vi "ParameterUpdate.vi"(5 "模式":T1(ring)=enum."updatesave", 7 "productsName":string, 8 "limitL":dbl=nan, 9 "limitH":dbl=nan, 10 "vaule":dbl=nan, 11 "parameterName":string) -> ()   [LabVIEW 2012]
uses:
  <vilib>/Utility/VariantDataType/Type.ctl
  <vilib>/Utility/VariantDataType/VariantType.lvlib
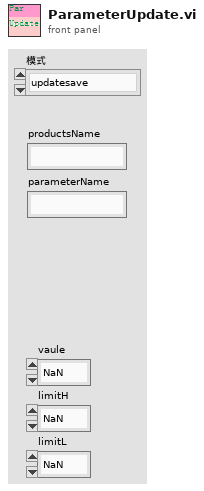
[diagram p1: front panel]
types:
  T1 = enum16{"updatedata", "updatesave", "updateresult", "updateresultempty"}
  T2 = typedef "VariantType.lvlib/Type.ctl" = enum8{"Invalid Type", "Void", "I8", "I16", "I32", "I64", "U8", "U16", "U32", "U64", "Single Float", "Double Float", "Extended Float", "Single Complex", "Double Complex", "Extended Complex", "Enum U8", "Enum U16", "Enum U32", "Enum U64", "Single Float With Unit", "Double Float With Unit", "Extended Float With Unit", "Single Complex with Unit", "Double Complex with Unit", "Extended Complex with Unit", "Boolean", "String", "Path", "Picture", "Tag", "Array", "Cluster", "Variant", "LV Variant", "Waveform", "Timestamp", "Digital Waveform", "Digital Data", "ExpressData", "Refnum", "External Data", "VI", "Poly VI", "LabVIEW Class Instance", "Fixed Point"}
  T3 = enum16{"selectdata", "selectsave", "selectlist", "selectshow"}
  T4 = cluster{"Type Enum":T2, "标签.文本":string, "productsName":string}
  T5 = cluster{"Type Enum":T2, "标签.文本":string, "productsName":string}[]
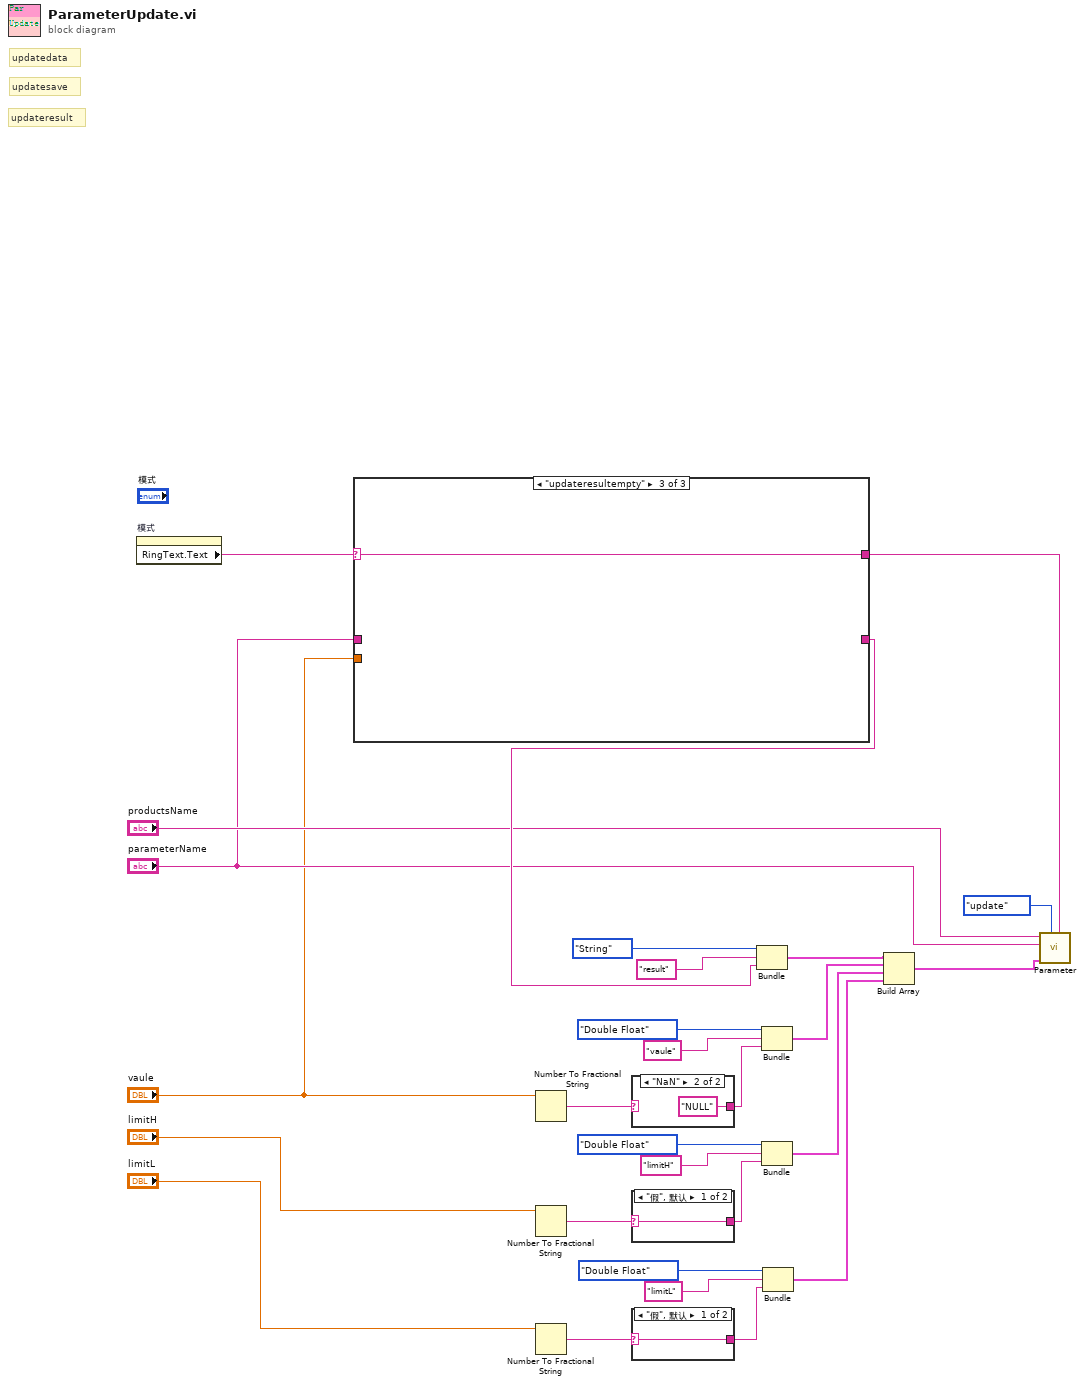
[diagram p0: block diagram]
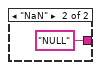
[diagram p3: hidden frame]
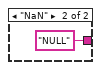
[diagram p4: hidden frame]
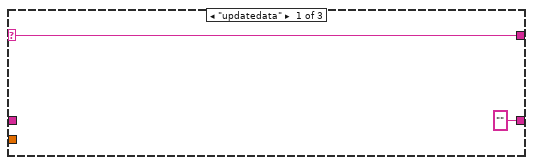
[diagram p5: hidden frame]
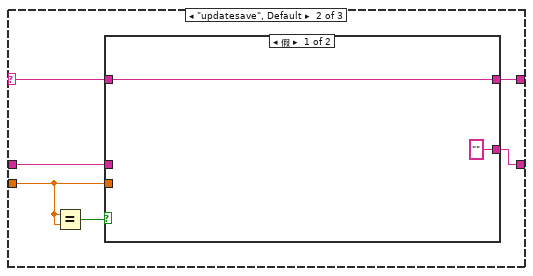
[diagram p6: hidden frame]
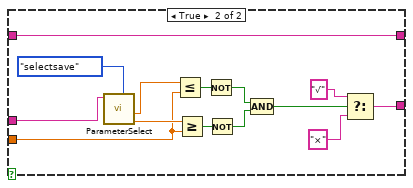
[diagram p7: hidden frame]
diagram:
  # "updatedata"
  # "updatesave"
  # "updateresult"
  n1 = property on="模式" class="Enum (严格)"() -> ("RingText.Text"=w28:string)  [unwired: 2 in, 2 out]
  n2 = case shown="\"updateresultempty\"" w28 {
    selector: w28 -> [w30 w34 w53]
    tunnel: "parameterName" -> [_ w36 _]
    tunnel: ["" ("productsName") w35 _] -> w12
    tunnel: [w30 w33 w53] -> w13
    tunnel: "vaule" -> [_ w31 _]
    frame "updatedata" {
    }
    frame "updatesave", Default {
      n3 = Equal?(x=w31, y=w31) -> (x = y?=w32:bool)
      n4 = case shown="假" w32 {
        tunnel: w36 -> [_ w52]
        tunnel: ["" ("productsName") w48] -> w35
        tunnel: w31 -> [_ w41]
        tunnel: w34 -> [w38 w39]
        tunnel: [w38 w39] -> w33
        frame False {
        }
        frame True {
          n5 = call "ParameterSelect.vi"("模式"=T3."selectsave", "parameterName"=w52) -> ("limitL"=w43:dbl, "limitH"=w42:dbl)  [unwired: 4 in, 4 out]
          n6 = Less Or Equal?(x=w42, y=w41) -> (x <= y?=w47:bool)
          n7 = Greater Or Equal?(x=w43, y=w41) -> (x >= y?=w45:bool)
          n8 = Not(x=w47) -> (.not. x?=w46:bool)
          n9 = Not(x=w45) -> (.not. x?=w44:bool)
          n10 = Compound Arithmetic op=AND(w46, w44) -> (w40:bool)
          n11 = Select(t="√" ("productsName"), s=w40, f="×" ("productsName")) -> (s? t:f=w48:string)
        }
      }
    }
    frame "updateresultempty" {
    }
  }
  n12 = Number To Fractional String(number="vaule") -> (F-format string=w8:string)  [unwired: 3 in]
  n13 = Number To Fractional String(number="limitH") -> (F-format string=w17:string)  [unwired: 3 in]
  n14 = Number To Fractional String(number="limitL") -> (F-format string=w19:string)  [unwired: 3 in]
  n15 = case shown="\"NaN\"" w8 {
    selector: w8 -> [w54 _]
    tunnel: [w54 "NULL"] -> w9
    frame "假", Default {
    }
    frame "NaN" {
    }
  }
  n16 = case shown="\"假\", 默认" w17 {
    selector: w17 -> [w56 _]
    tunnel: [w56 "NULL"] -> w16
    frame "假", Default {
    }
    frame "NaN" {
    }
  }
  n17 = case shown="\"假\", 默认" w19 {
    selector: w19 -> [w58 _]
    tunnel: [w58 "NULL"] -> w18
    frame "假", Default {
    }
    frame "NaN" {
    }
  }
  n18 = Bundle("Type Enum"=Type."String", "标签.文本"="result", "productsName"=w12) -> (w4:T4)  [unwired: 1 in]
  n19 = Bundle("Type Enum"=Type."Double Float", "标签.文本"="vaule", w9) -> (w5:cluster{"Type Enum":T2, "标签.文本":string, string})  [unwired: 1 in]
  n20 = Bundle("Type Enum"=Type."Double Float", "标签.文本"="limitH", w16) -> (w21:cluster{"Type Enum":T2, "标签.文本":string, string})  [unwired: 1 in]
  n21 = Bundle("Type Enum"=Type."Double Float", "标签.文本"="limitL", w18) -> (w20:cluster{"Type Enum":T2, "标签.文本":string, string})  [unwired: 1 in]
  n22 = Build Array(w4, w5, w21, w20) -> (w15:T5)
  n23 = call "Parameter.vi"("继承模式"=w13, "模式"=enum16{"select", "insert", "update", "delete"}."update", "nameData"=w15, "parameterName"="parameterName", "productsName"="productsName") -> ()  [unwired: 6 in, 1 out]
